vi "Facade.vi"(0 "Data In":T5={"Type"=enum."Lowpass", "CF (kHz)"=0.0, "BW (kHz)"=0.0, "Cascade"=FALSE, "Quadrature"=FALSE, "Scale Factor"=0.0, "Stages"=[], "Class"=enum."Elliptic", "Order"=0, "BWUnits"=enum."Linear"} {"Stages"."IIR Filter"."Forward Coefficients" format="%.4f"; "Stages"."IIR Filter"."Reverse Coefficients" format="%.4f"}, 2 "Display State In":T3, 3 "Container State":T4) -> (6 "Data Out":T5={"Type"=enum."Lowpass", "CF (kHz)"=0.0, "BW (kHz)"=0.0, "Cascade"=FALSE, "Quadrature"=FALSE, "Scale Factor"=0.0, "Stages"=[], "Class"=enum."Elliptic", "Order"=0, "BWUnits"=enum."Linear"} {"Stages"."IIR Filter"."Forward Coefficients" format="%.4f"; "Stages"."IIR Filter"."Reverse Coefficients" format="%.4f"}, 7 "Display State Out":T3, 8 "Action":T2)   [LabVIEW 2020, in "Filter (G3).xctl"]
uses:
  Filter (G3).xctl
  Filter Data.ctl
  Filter Type.ctl
  Filter VIs/Filter-Bandwidth Units.ctl
  <vilib>/_xctls/Container State.ctl
  State.ctl
  <vilib>/_xctls/Action.ctl
  <vilib>/_xctls/XControlSupport.lvlib
panel:
  in  "BWUnits":u16(ring) caption="Filter" items=["kHz", "Octaves", "Min-Max"]
  in  "Cascade":bool
  in  "F2":dbl caption="BW"
  in  "Type":T1(ring) caption="Filter"
  in  "F1":dbl caption="CF (kHz)"
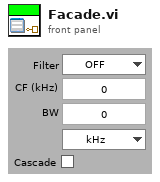
[diagram p1: front panel]
types:
  T1 = enum16{"OFF", "Lowpass", "Highpass", "Bandpass", "Bandstop"}
  T2 = typedef "XControlSupport.lvlib/Action.ctl" = cluster{"Data Changed?":bool, "State Changed?":bool, "Action Name":string}
  T3 = typedef "Filter (G3).xctl/State.ctl" = cluster{"Show cascade":bool, "Label color":u32, "TypeRef":refnum<vi>, "UnitsRef":refnum<vi>, "actions":string[]}
  T4 = typedef "XControlSupport.lvlib/Container State.ctl" = cluster{"Indicator?":bool, "Run Mode?":bool, " Refnum":refnum<vi>}
  T5 = typedef "Filter (G3).xctl/Filter Data.ctl" = cluster{"Type":T6, "CF (kHz)":dbl, "BW (kHz)":dbl, "Cascade":bool, "Quadrature":bool, "Scale Factor":dbl, "Stages":cluster{"IIR Filter":cluster{"filter structure":enum32{"IIR 2nd Order", "IIR 4th Order"}, "Reverse Coefficients":dbl[], "Forward Coefficients":dbl[]}, "State":dbl[]}[], "Class":enum16{"Elliptic", "Butterworth"}, "Order":i32, "BWUnits":T7}
  T6 = typedef "Filter (G3).xctl/Filter Type.ctl" = enum16{"OFF", "Lowpass", "Highpass", "Bandpass", "Bandstop"}
  T7 = typedef "Filter-Bandwidth Units.ctl" = enum16{"Linear", "Octaves", "Min-Max"}
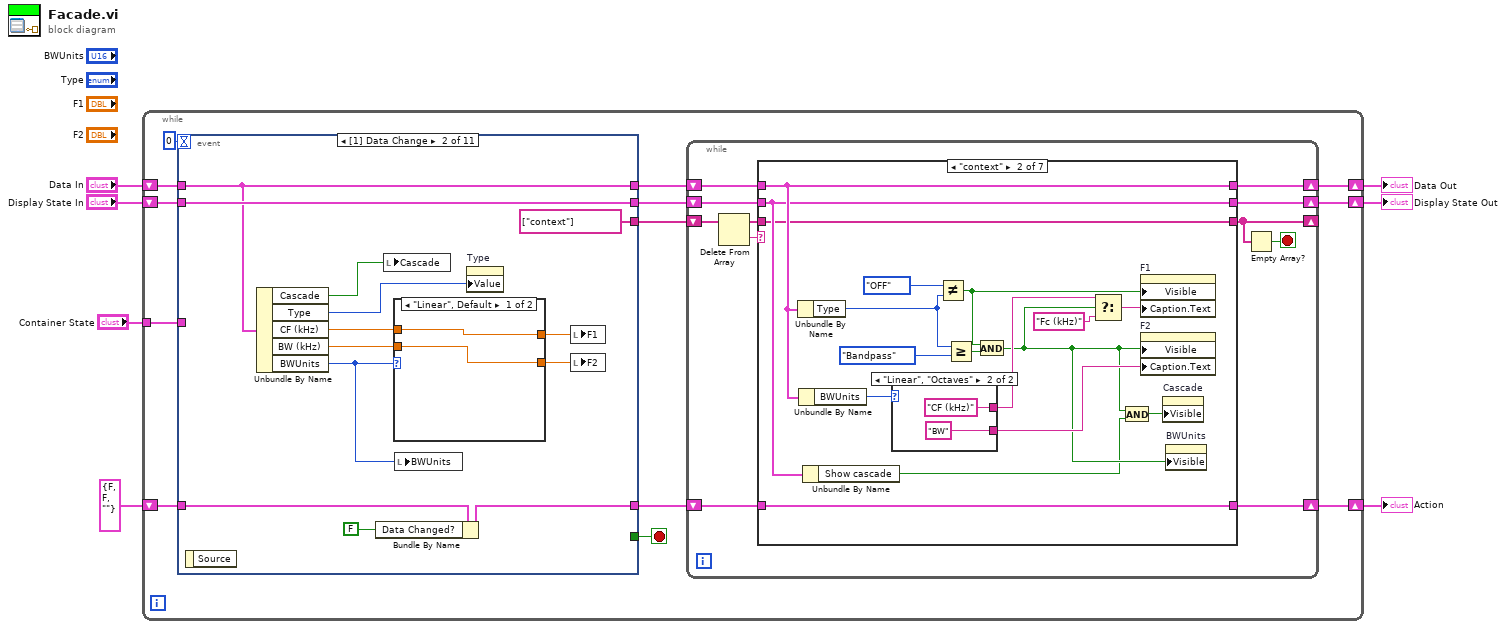
[diagram p0: block diagram]
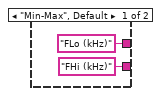
[diagram p3: hidden frame]
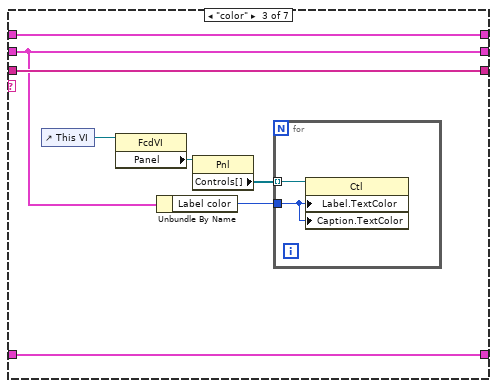
[diagram p4: hidden frame]
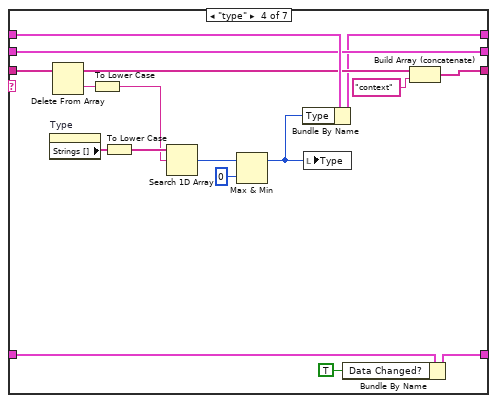
[diagram p5: hidden frame]
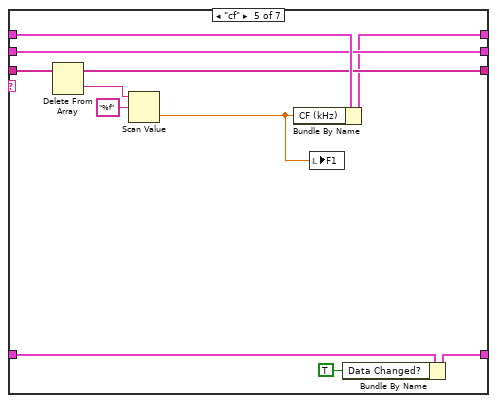
[diagram p6: hidden frame]
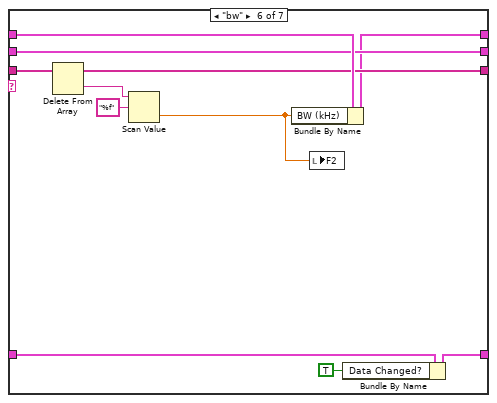
[diagram p7: hidden frame]
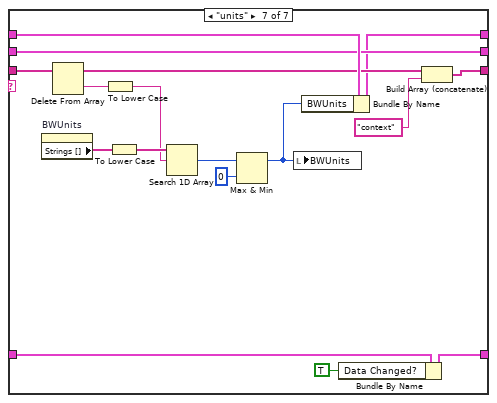
[diagram p8: hidden frame]
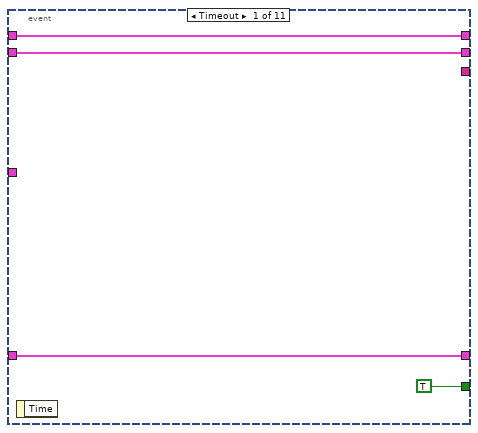
[diagram p9: hidden frame]
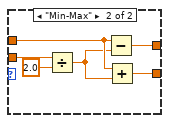
[diagram p10: hidden frame]
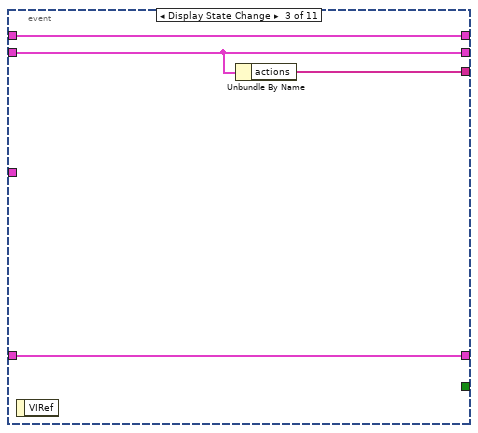
[diagram p11: hidden frame]
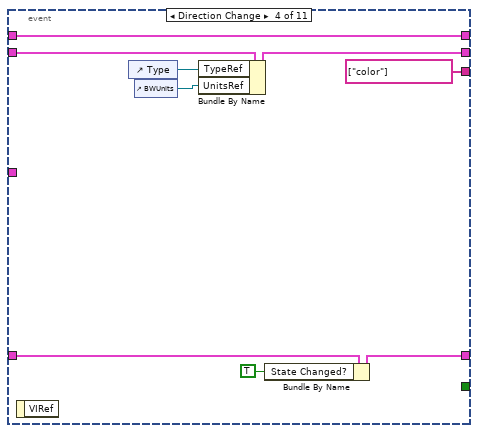
[diagram p12: hidden frame]
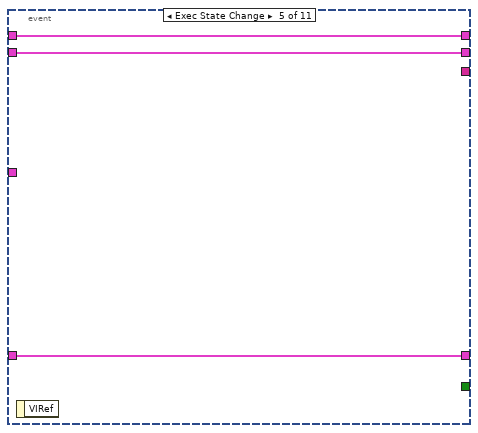
[diagram p13: hidden frame]
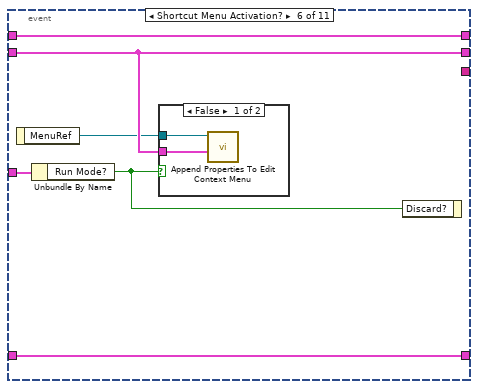
[diagram p14: hidden frame]
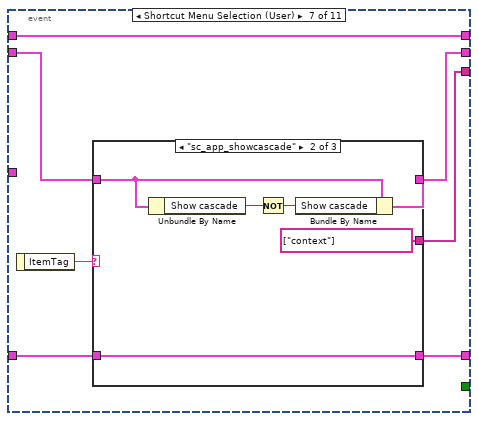
[diagram p16: hidden frame]
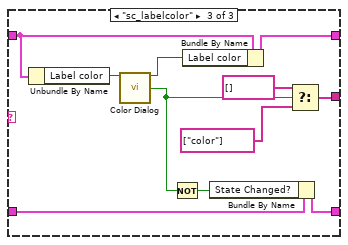
[diagram p18: hidden frame]
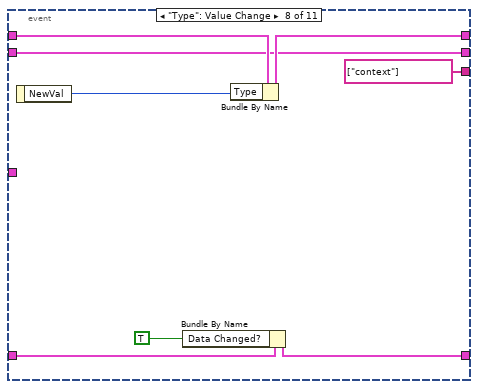
[diagram p19: hidden frame]
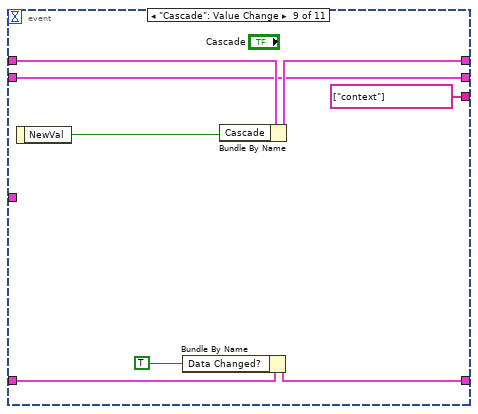
[diagram p20: hidden frame]
diagram:
  n1 = while {
    shift-right: [w12] -> w4
    shift-left: "Display State In" -> [w20]
    tunnel: "Container State" -> [w10]
    shift-right: [w13] -> w7
    shift-left: "Data In" -> [w17]
    shift-right: [w8] -> w2
    shift-left: T2 {"Data Changed?"=FALSE, "State Changed?"=FALSE, "Action Name"=""} ("Action") -> [w16]
    stop <- w19 stop-if-true
    n2 = event shown="[1] Data Change" {
      selector: _ -> [_ _ _ _ _ _ _ _ _ _ _]
      dyn-events: _ -> [_ _ _ _ _ _ _ _ _ _ _]
      timeout: 0 -> [_ _ _ _ _ _ _ _ _ _ _]
      tunnel: w20 -> [w124 w131 w149 w160 w163 w166 w177 w201 w209 w221 w244]
      tunnel: [w124 w131 w149 w156 w163 w166 w175 w201 w209 w221 w244] -> w15
      tunnel: [TRUE _ _ _ _ _ _ _ _ _ _] -> w19
      tunnel: w10 -> [_ _ _ _ _ w167 _ _ _ _ _]
      tunnel: w17 -> [w123 w130 w151 w159 w162 w169 w178 w205 w213 w215 w238]
      tunnel: [w123 w130 w151 w159 w162 w169 w178 w204 w212 w225 w248] -> w14
      tunnel: [w125 w138 w150 w153 w161 w168 w172 w202 w210 w222 w245] -> w9
      tunnel: w16 -> [w125 w139 w150 w158 w161 w168 w173 w203 w211 w224 w247]
      tunnel: [_ string[] ["context"] w148 string[] ["color"] _ _ w174 string[] ["context"] string[] ["context"] _ string[] ["context"]] -> w11
      event Timeout {
        n3 = event-data() -> ()  [unwired: 1 in, 1 out]
      }
      event Data Change {
        n4 = event-data() -> ()  [unwired: 1 in, 1 out]
        n5 = Unbundle By Name(w130) -> ("Cascade"=w129:bool, "Type"=w132:T6, "CF (kHz)"=w136:dbl, "BW (kHz)"=w134:dbl, "BWUnits"=w127:T7)
        n6 = Bundle By Name(cluster=w139, "Data Changed?"=FALSE) -> (w138:T2)
        n7 = local write "Cascade"(w129) -> ()
        n8 = case shown="\"Linear\", Default" w127 {
          tunnel: w136 -> [w141 w144]
          tunnel: [w141 w145] -> w135
          tunnel: [w140 w142] -> w133
          tunnel: w134 -> [w140 w147]
          frame "Linear", Default {
          }
          frame "Min-Max" {
            n9 = Divide(x=w147, y=2.0) -> (x/y=w143:dbl)
            n10 = Subtract(x=w144, y=w143) -> (x-y=w145:dbl)
            n11 = Add(x=w144, y=w143) -> (x+y=w142:dbl)
          }
        }
        n12 = local write "BWUnits"(w127) -> ()
        n13 = property on="Type" class="Enum (strict)"("Value"=w132) -> ()  [unwired: 2 in, 2 out]
        n14 = local write "F1"(w135) -> ()
        n15 = local write "F2"(w133) -> ()
      }
      event Display State Change {
        n16 = event-data() -> ()  [unwired: 1 in, 1 out]
        n17 = Unbundle By Name(w149) -> ("actions"=w148:string[])
      }
      event Direction Change {
        n18 = event-data() -> ()  [unwired: 1 in, 1 out]
        n19 = control-ref of="Type"() -> (w155:refnum<vi>)
        n20 = control-ref of="BWUnits"() -> (w154:refnum<vi>)
        n21 = Bundle By Name(cluster=w160, "TypeRef"=w155, "UnitsRef"=w154) -> (w156:T3)
        n22 = Bundle By Name(cluster=w158, "State Changed?"=TRUE) -> (w153:T2)
      }
      event Exec State Change {
        n23 = event-data() -> ()  [unwired: 1 in, 1 out]
      }
      event Shortcut Menu Activation? {
        n24 = event-data() -> ("MenuRef"=w164:refnum<k9>)  [unwired: 1 in]
        n25 = Unbundle By Name(w167) -> ("Run Mode?"=w165:bool)
        n26 = case shown="False" w165 {
          tunnel: w166 -> [w171 _]
          tunnel: w164 -> [w170 _]
          frame False {
            n27 = call "Append Properties To Edit Context Menu.vi"("State"=w171, "Menu in"=w170) -> ()  [unwired: 10 in]
          }
          frame True {
          }
        }
        n28 = event-data("Discard?"=w165) -> ()  [unwired: 1 in, 1 out]
      }
      event Shortcut Menu Selection (User) {
        n29 = event-data() -> ("ItemTag"=w176:string)  [unwired: 1 in]
        n30 = case shown="\"sc_app_showcascade\"" w176 {
          tunnel: w177 -> [w180 w186 w197]
          tunnel: [w180 w185 w192] -> w175
          tunnel: [_ string[] ["context"] w190] -> w174
          tunnel: w173 -> [w179 w181 w195]
          tunnel: [w179 w181 w194] -> w172
          frame "False", Default {
          }
          frame "sc_app_showcascade" {
            n31 = Unbundle By Name(w186) -> ("Show cascade"=w184:bool)
            n32 = Not(x=w184) -> (.not. x?=w183:bool)
            n33 = Bundle By Name(cluster=w186, "Show cascade"=w183) -> (w185:T3)
          }
          frame "sc_labelcolor" {
            n34 = Unbundle By Name(w197) -> ("Label color"=w196:u32)
            n35 = call "Color Dialog.vi"("Color in"=w196) -> ("Color out"=w191:u32, "Canceled?"=w189:bool)  [unwired: 13 in]
            n36 = Not(x=w189) -> (.not. x?=w193:bool)
            n37 = Bundle By Name(cluster=w197, "Label color"=w191) -> (w192:T3)
            n38 = Bundle By Name(cluster=w195, "State Changed?"=w193) -> (w194:T2)
            n39 = Select(t=string[] [], s=w189, f=string[] ["color"]) -> (s? t:f=w190:string[])
          }
        }
      }
      event "Type": Value Change {
        n40 = event-data() -> ("NewVal"=w200:T1)  [unwired: 1 in]
        n41 = Bundle By Name(cluster=w203, "Data Changed?"=TRUE) -> (w202:T2)
        n42 = Bundle By Name(cluster=w205, "Type"=w200) -> (w204:T5)
      }
      event "Cascade": Value Change {
        n43 = event-data() -> ("NewVal"=w208:bool)  [unwired: 1 in]
        n44 = Bundle By Name(cluster=w211, "Data Changed?"=TRUE) -> (w210:T2)
        n45 = Bundle By Name(cluster=w213, "Cascade"=w208) -> (w212:T5)
      }
      event "F1", "F2": Value Change {
        n46 = event-data() -> ()  [unwired: 1 in, 1 out]
        n47 = local read "BWUnits"() -> (w214:u16)
        n48 = local read "F1"() -> (w220:dbl)
        n49 = local read "F2"() -> (w218:dbl)
        n50 = case shown="2" w214 {
          selector: w214 -> [w226 w229]
          tunnel: w220 -> [w228 w232]
          tunnel: [w228 w234] -> w219
          tunnel: [w227 w230] -> w217
          tunnel: w218 -> [w227 w231]
          tunnel: [w226 w229] -> w216
          frame 0, Default {
          }
          frame 2 {
            n51 = Add(x=w232, y=w231) -> (x+y=w235:dbl)
            n52 = Subtract(x=w231, y=w232) -> (x-y=w230:dbl)
            n53 = Divide(x=w235, y=2.0) -> (x/y=w234:dbl)
          }
        }
        n54 = Bundle By Name(cluster=w224, "Data Changed?"=TRUE) -> (w222:T2)
        n55 = Bundle By Name(cluster=w215, "CF (kHz)"=w219, "BW (kHz)"=w217, "BWUnits"=w216) -> (w225:T5)
      }
      event "BWUnits": Value Change {
        n56 = event-data() -> ()  [unwired: 1 in, 1 out]
        n57 = local read "BWUnits"() -> (w237:u16)
        n58 = local read "F1"() -> (w243:dbl)
        n59 = local read "F2"() -> (w241:dbl)
        n60 = case shown="2" w237 {
          selector: w237 -> [w249 w252]
          tunnel: w243 -> [w251 w255]
          tunnel: [w251 w257] -> w242
          tunnel: [w250 w253] -> w240
          tunnel: w241 -> [w250 w254]
          tunnel: [w249 w252] -> w239
          frame 0, Default {
          }
          frame 2 {
            n61 = Add(x=w255, y=w254) -> (x+y=w258:dbl)
            n62 = Subtract(x=w254, y=w255) -> (x-y=w253:dbl)
            n63 = Divide(x=w258, y=2.0) -> (x/y=w257:dbl)
          }
        }
        n64 = Bundle By Name(cluster=w247, "Data Changed?"=TRUE) -> (w245:T2)
        n65 = Bundle By Name(cluster=w238, "CF (kHz)"=w242, "BW (kHz)"=w240, "BWUnits"=w239) -> (w248:T5)
      }
    }
    n66 = while {
      shift-right: [w25] -> _
      shift-left: w11 -> [w27]
      shift-right: [w21] -> w8
      shift-left: w9 -> [w22]
      shift-right: [w29] -> w13
      shift-left: w14 -> [w31]
      shift-right: [w28] -> w12
      shift-left: w15 -> [w30]
      stop <- w24 stop-if-true
      n67 = Delete From Array(array=w27) -> (deleted portion=w23:string, array with subset deleted=w26:string[])  [unwired: 2 in]
      n68 = case shown="\"context\"" w23 {
        tunnel: w31 -> [w35 w39 w64 w83 w94 w105 w122]
        tunnel: w30 -> [w34 w38 w59 w82 w93 w104 w121]
        tunnel: [w35 w39 w64 w74 w89 w100 w113] -> w29
        tunnel: [w34 w38 w59 w82 w93 w104 w121] -> w28
        tunnel: w26 -> [w33 w37 w63 w80 w91 w102 w119]
        tunnel: [w33 w37 w63 w70 w90 w101 w109] -> w25
        tunnel: w22 -> [w32 w36 w57 w81 w92 w103 w120]
        tunnel: [w32 w36 w57 w72 w88 w99 w111] -> w21
        frame "", Default {
        }
        frame "context" {
          n69 = Unbundle By Name(w39) -> ("Type"=w47:T6)
          n70 = Unbundle By Name(w39) -> ("BWUnits"=w40:T7)
          n71 = Unbundle By Name(w38) -> ("Show cascade"=w41:bool)
          n72 = case shown="\"Linear\", \"Octaves\"" w40 {
            tunnel: ["FLo (kHz)" "CF (kHz)"] -> w49
            tunnel: ["FHi (kHz)" "BW"] -> w46
            frame "Min-Max", Default {
            }
            frame "Linear", "Octaves" {
            }
          }
          n73 = Not Equal?(x=Filter_Type."OFF" ("Type"), y=w47) -> (x != y?=w51:bool)
          n74 = Greater Or Equal?(x=w47, y=Filter_Type."Bandpass" ("Type")) -> (x >= y?=w52:bool)
          n75 = And(x=w51, y=w52) -> (x .and. y?=w45:bool)
          n76 = Select(t=w49, s=w45, f="Fc (kHz)" ("t")) -> (s? t:f=w50:string)
          n77 = And(x=w45, y=w41) -> (x .and. y?=w42:bool)
          n78 = property on="F1" class="DigNum (strict)"("Visible"=w51, "Caption.Text"=w50) -> ()  [unwired: 2 in, 2 out]
          n79 = property on="F2" class="DigNum (strict)"("Visible"=w45, "Caption.Text"=w46) -> ()  [unwired: 2 in, 2 out]
          n80 = property on="Cascade" class="Bool (strict)"("Visible"=w42) -> ()  [unwired: 2 in, 2 out]
          n81 = property on="BWUnits" class="Ring (strict)"("Visible"=w45) -> ()  [unwired: 2 in, 2 out]
        }
        frame "color" {
          n82 = control-ref of="This VI"() -> (w62:refnum<vi>)
          n83 = property on="Property Node" class="FcdVI"(reference=w62) -> ("Panel"=w61:refnum<vi>)  [unwired: 1 in, 2 out]
          n84 = Unbundle By Name(w59) -> ("Label color"=w58:u32)
          n85 = property class="Pnl"(reference=w61) -> ("Controls[]"=w60:refnum<vi>[])  [unwired: 1 in, 2 out]
          n86 = for {
            tunnel: w60 -> [w66] mode=indexing
            tunnel: w58 -> [w65]
            n87 = property class="Ctl"(reference=w66, "Label.TextColor"=w65, "Caption.TextColor"=w65) -> ()  [unwired: 1 in, 2 out]
          }
        }
        frame "type" {
          n88 = property on="Type" class="Enum (strict)"() -> ("Strings []"=w78:string[])  [unwired: 2 in, 2 out]
          n89 = Delete From Array(array=w80) -> (deleted portion=w77:string, array with subset deleted=w79:string[])  [unwired: 2 in]
          n90 = To Lower Case(string=w77) -> (all lower case string=w67:string)
          n91 = To Lower Case(string=w78) -> (all lower case string=w68:string[])
          n92 = Search 1D Array(1D array=w68, element=w67) -> (index of element=w76:i32)  [unwired: 1 in]
          n93 = Max & Min(x=w76, y=0) -> (max(x,y)=w73:i32)  [unwired: 1 out]
          n94 = Bundle By Name(cluster=w83, "Type"=w73) -> (w74:T5)
          n95 = local write "Type"(w73) -> ()
          n96 = Bundle By Name(cluster=w81, "Data Changed?"=TRUE) -> (w72:T2)
          n97 = Build Array (concatenate)(w79, "context") -> (w70:string[])
        }
        frame "cf" {
          n98 = Delete From Array(array=w91) -> (deleted portion=w86:string, array with subset deleted=w90:string[])  [unwired: 2 in]
          n99 = Scan Value(string=w86, format string="%f") -> (value=w85:dbl)  [unwired: 1 in, 1 out]
          n100 = Bundle By Name(cluster=w94, "CF (kHz)"=w85) -> (w89:T5)
          n101 = local write "F1"(w85) -> ()
          n102 = Bundle By Name(cluster=w92, "Data Changed?"=TRUE) -> (w88:T2)
        }
        frame "bw" {
          n103 = Delete From Array(array=w102) -> (deleted portion=w97:string, array with subset deleted=w101:string[])  [unwired: 2 in]
          n104 = Scan Value(string=w97, format string="%f") -> (value=w96:dbl)  [unwired: 1 in, 1 out]
          n105 = Bundle By Name(cluster=w105, "BW (kHz)"=w96) -> (w100:T5)
          n106 = local write "F2"(w96) -> ()
          n107 = Bundle By Name(cluster=w103, "Data Changed?"=TRUE) -> (w99:T2)
        }
        frame "units" {
          n108 = property on="BWUnits" class="Ring (strict)"() -> ("Strings []"=w117:string[])  [unwired: 2 in, 2 out]
          n109 = Delete From Array(array=w119) -> (deleted portion=w116:string, array with subset deleted=w118:string[])  [unwired: 2 in]
          n110 = To Lower Case(string=w116) -> (all lower case string=w106:string)
          n111 = To Lower Case(string=w117) -> (all lower case string=w107:string[])
          n112 = Search 1D Array(1D array=w107, element=w106) -> (index of element=w115:i32)  [unwired: 1 in]
          n113 = Max & Min(x=w115, y=0) -> (max(x,y)=w112:i32)  [unwired: 1 out]
          n114 = local write "BWUnits"(w112) -> ()
          n115 = Bundle By Name(cluster=w122, "BWUnits"=w112) -> (w113:T5)
          n116 = Bundle By Name(cluster=w120, "Data Changed?"=TRUE) -> (w111:T2)
          n117 = Build Array (concatenate)(w118, "context") -> (w109:string[])
        }
      }
      n118 = Empty Array?(array=w25) -> (empty?=w24:bool)
    }
  }
  "Display State Out" <- w4
  "Data Out" <- w7
  "Action" <- w2
